vi "deleteFile.vi"(8 "error in (no error)":errorcluster caption="entrée d'erreur (pas d'erreur)", 11 "Python en entrée":refnum<class "Python.lvclass">) -> (0 "error out":errorcluster caption="sortie d'erreur", 3 "Python en sortie":refnum<class "Python.lvclass">)   [LabVIEW 2020, in "Python.lvclass"]
uses:
  Python.lvclass
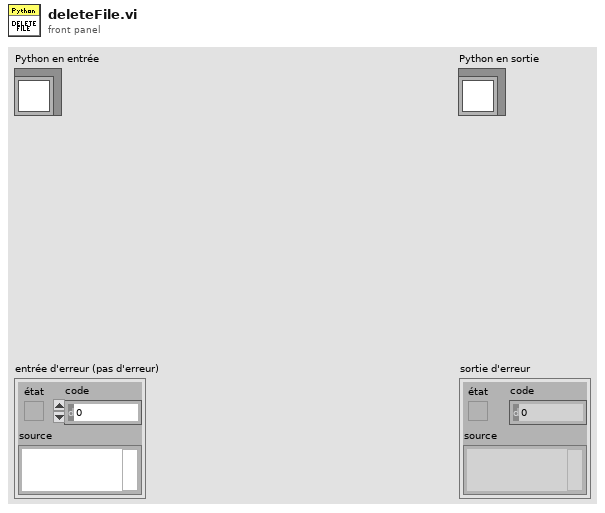
[diagram p1: front panel]
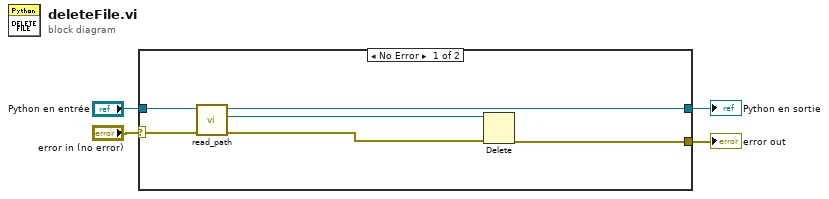
[diagram p0: block diagram]
diagram:
  n1 = case shown="No Error" "error in (no error)" {
    selector: "error in (no error)" -> [w8 w12]
    tunnel: [w5 w12] -> w3
    tunnel: [w9 w11] -> w1
    tunnel: "Python en entrée" -> [w10 w11]
    frame No Error {
      n2 = call-dynamic "read_path.vi"("error in (no error)"=w8, "Python en entrée"=w10) -> ("error out"=w6:errorcluster, "chemin"=w7:path, "Python en sortie"=w9:refnum<class "Python.lvclass">)  [unwired: 7 in]
      n3 = Delete(path (use dialog)=w7, error in=w6) -> (error out=w5:errorcluster)  [unwired: 3 in, 2 out]
    }
    frame Error {
    }
  }
  "error out" <- w3
  "Python en sortie" <- w1
